vi "Register gRPC Methods.vi"(8 "error in (no error)":errorcluster, 11 "gRPC service in":refnum<class "Manager.lvclass">) -> (0 "error out":errorcluster, 3 "gRPC service out":refnum<class "Manager.lvclass">)   [LabVIEW 2021, in "CIF_Manager_server.lvlib" / "Manager.lvclass"]
uses:
  Manager.lvclass
  typeDefs/Server Internal UEs.ctl
  typeDefs/Server Internal Message.ctl
  typeDefs/Server gRPC UEs.ctl
  <vilib>/gRPC/LabVIEW gRPC Library/Server API/typeDefs/gRPCId Cluster.ctl
  <vilib>/gRPC/LabVIEW gRPC Library/Shared/grpcId.ctl
  Manager.lvclass/Manager.ctl
  <vilib>/gRPC/LabVIEW gRPC Library/grpc-lvsupport-release.lvlib
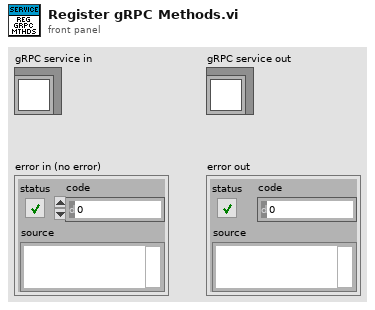
[diagram p1: front panel]
types:
  T1 = typedef "CIF_Manager_server.lvlib/Manager.lvclass/Server gRPC UEs.ctl" = cluster{"Manager LoadPlugin gRPC UE":refnum<user-event>, "Manager RegisterPlugin gRPC UE":refnum<user-event>, "Manager UnregisterPlugin gRPC UE":refnum<user-event>, "Manager QueryPluginTypes gRPC UE":refnum<user-event>, "Manager AbortPlugin gRPC UE":refnum<user-event>, "Manager UnloadAllPlugins gRPC UE":refnum<user-event>, "Manager Destroy gRPC UE":refnum<user-event>, "Manager Ping gRPC UE":refnum<user-event>, "Manager QueryErrors gRPC UE":refnum<user-event>, "Manager QueryConfig gRPC UE":refnum<user-event>, "Manager QueryInfo gRPC UE":refnum<user-event>, "Manager ResetErrorIndex gRPC UE":refnum<user-event>, "Manager ResetConfigIndex gRPC UE":refnum<user-event>, "Manager ResetInfoIndex gRPC UE":refnum<user-event>, "Manager QueryPluginInfo gRPC UE":refnum<user-event>, "Manager QueryPlugin gRPC UE":refnum<user-event>, "Manager QuerySystemStatus gRPC UE":refnum<user-event>, "Manager UpdateClock gRPC UE":refnum<user-event>, "Manager CreateOrch gRPC UE":refnum<user-event>, "Manager QueryClockStatus gRPC UE":refnum<user-event>, "Manager QueryAllChannels gRPC UE":refnum<user-event>, "Manager RegisterPluginLoader gRPC UE":refnum<user-event>, "Manager UnregisterPluginLoader gRPC UE":refnum<user-event>, "Manager CreatePluginLoader gRPC UE":refnum<user-event>, "Manager DestroyPluginLoader gRPC UE":refnum<user-event>, "Manager QueryPluginLoaders gRPC UE":refnum<user-event>}
  T2 = typedef "CIF_Manager_server.lvlib/Manager.lvclass/Server Internal UEs.ctl" = cluster{"Manager LoadPlugin Internal UE":refnum<user-event>, "Manager RegisterPlugin Internal UE":refnum<user-event>, "Manager UnregisterPlugin Internal UE":refnum<user-event>, "Manager QueryPluginTypes Internal UE":refnum<user-event>, "Manager AbortPlugin Internal UE":refnum<user-event>, "Manager UnloadAllPlugins Internal UE":refnum<user-event>, "Manager Destroy Internal UE":refnum<user-event>, "Manager Ping Internal UE":refnum<user-event>, "Manager QueryErrors Internal UE":refnum<user-event>, "Manager QueryConfig Internal UE":refnum<user-event>, "Manager QueryInfo Internal UE":refnum<user-event>, "Manager ResetErrorIndex Internal UE":refnum<user-event>, "Manager ResetConfigIndex Internal UE":refnum<user-event>, "Manager ResetInfoIndex Internal UE":refnum<user-event>, "Manager QueryPluginInfo Internal UE":refnum<user-event>, "Manager QueryPlugin Internal UE":refnum<user-event>, "Manager QuerySystemStatus Internal UE":refnum<user-event>, "Manager UpdateClock Internal UE":refnum<user-event>, "Manager CreateOrch Internal UE":refnum<user-event>, "Manager QueryClockStatus Internal UE":refnum<user-event>, "Manager QueryAllChannels Internal UE":refnum<user-event>, "Manager RegisterPluginLoader Internal UE":refnum<user-event>, "Manager UnregisterPluginLoader Internal UE":refnum<user-event>, "Manager CreatePluginLoader Internal UE":refnum<user-event>, "Manager DestroyPluginLoader Internal UE":refnum<user-event>, "Manager QueryPluginLoaders Internal UE":refnum<user-event>}
  T3 = typedef "grpc-lvsupport-release.lvlib/grpcId.ctl" = u64
  T4 = typedef "CIF_Manager_server.lvlib/Manager.lvclass/Server Internal Message UE.ctl" = refnum<user-event>
  T5 = typedef "grpc-lvsupport-release.lvlib/gRPCId Cluster UE.ctl" = refnum<user-event>
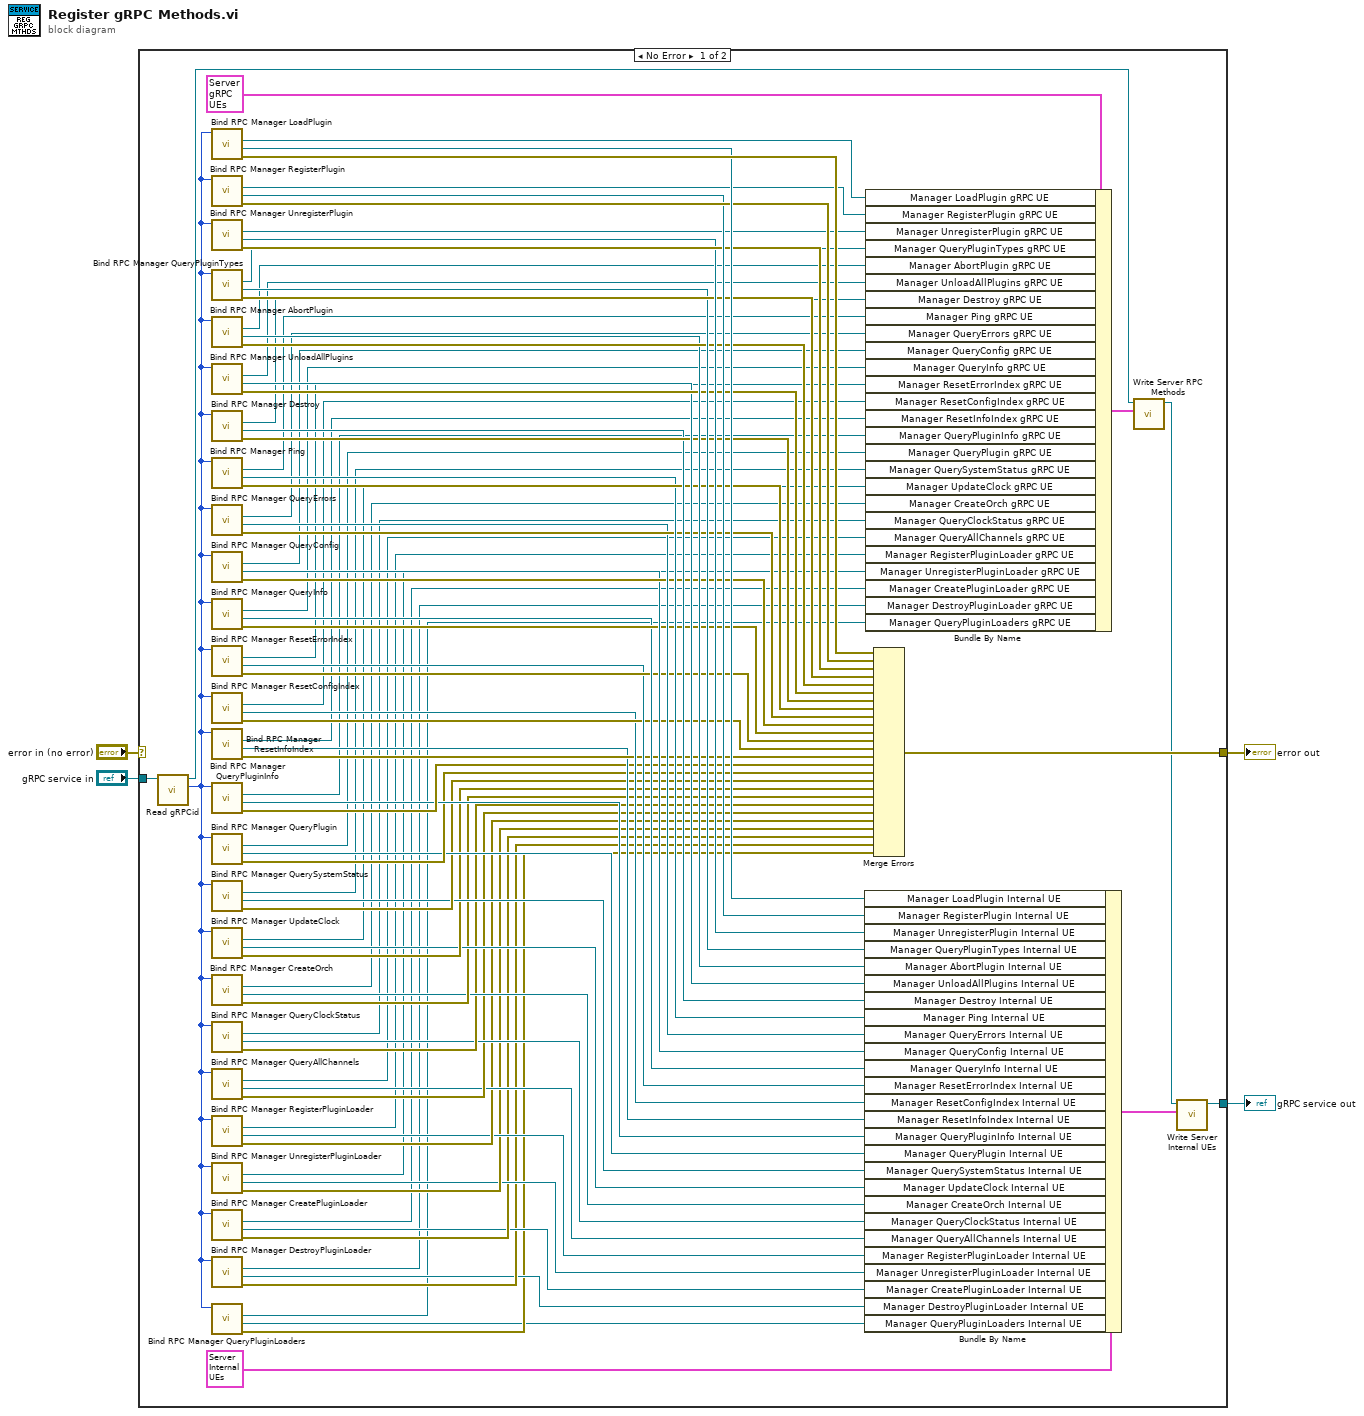
[diagram p0: block diagram]
diagram:
  n1 = case shown="No Error" "error in (no error)" {
    selector: "error in (no error)" -> [_ w93]
    tunnel: "gRPC service in" -> [w84 w94]
    tunnel: [w92 w93] -> w3
    tunnel: [w91 w94] -> w2
    frame No Error {
      n2 = call-dynamic "Read gRPCid.vi"("gRPC service in"=w84) -> ("gRPCid"=w83:T3, "gRPC service out"=w85:refnum<class "Manager.lvclass">)  [unwired: 8 in, 1 out]
      n3 = call "Bind RPC Manager LoadPlugin.vi"("gRPCid server in"=w83) -> ("error out"=w82:errorcluster, "Manager LoadPlugin Internal UE"=w81:T4, "Manager LoadPlugin gRPC UE"=w80:T5)  [unwired: 7 in, 1 out]
      n4 = call "Bind RPC Manager RegisterPlugin.vi"("gRPCid server in"=w83) -> ("error out"=w79:errorcluster, "Manager RegisterPlugin Internal UE"=w77:T4, "Manager RegisterPlugin gRPC UE"=w78:T5)  [unwired: 7 in, 1 out]
      n5 = call "Bind RPC Manager UnregisterPlugin.vi"("gRPCid server in"=w83) -> ("error out"=w76:errorcluster, "Manager UnregisterPlugin Internal UE"=w75:T4, "Manager UnregisterPlugin gRPC UE"=w74:T5)  [unwired: 7 in, 1 out]
      n6 = call "Bind RPC Manager QueryPluginTypes.vi"("gRPCid server in"=w83) -> ("error out"=w73:errorcluster, "Manager QueryPluginTypes Internal UE"=w71:T4, "Manager QueryPluginTypes gRPC UE"=w72:T5)  [unwired: 7 in, 1 out]
      n7 = call "Bind RPC Manager AbortPlugin.vi"("gRPCid server in"=w83) -> ("error out"=w70:errorcluster, "Manager AbortPlugin Internal UE"=w69:T4, "Manager AbortPlugin gRPC UE"=w68:T5)  [unwired: 7 in, 1 out]
      n8 = call "Bind RPC Manager UnloadAllPlugins.vi"("gRPCid server in"=w83) -> ("error out"=w67:errorcluster, "Manager UnloadAllPlugins Internal UE"=w65:T4, "Manager UnloadAllPlugins gRPC UE"=w66:T5)  [unwired: 7 in, 1 out]
      n9 = call "Bind RPC Manager Destroy.vi"("gRPCid server in"=w83) -> ("error out"=w64:errorcluster, "Manager Destroy Internal UE"=w63:T4, "Manager Destroy gRPC UE"=w62:T5)  [unwired: 7 in, 1 out]
      n10 = call "Bind RPC Manager Ping.vi"("gRPCid server in"=w83) -> ("error out"=w61:errorcluster, "Manager Ping Internal UE"=w59:T4, "Manager Ping gRPC UE"=w60:T5)  [unwired: 7 in, 1 out]
      n11 = call "Bind RPC Manager QueryErrors.vi"("gRPCid server in"=w83) -> ("error out"=w58:errorcluster, "Manager QueryErrors Internal UE"=w56:T4, "Manager QueryErrors gRPC UE"=w57:T5)  [unwired: 7 in, 1 out]
      n12 = call "Bind RPC Manager QueryConfig.vi"("gRPCid server in"=w83) -> ("error out"=w55:errorcluster, "Manager QueryConfig Internal UE"=w53:T4, "Manager QueryConfig gRPC UE"=w54:T5)  [unwired: 7 in, 1 out]
      n13 = call "Bind RPC Manager QueryInfo.vi"("gRPCid server in"=w83) -> ("error out"=w52:errorcluster, "Manager QueryInfo Internal UE"=w50:T4, "Manager QueryInfo gRPC UE"=w51:T5)  [unwired: 7 in, 1 out]
      n14 = call "Bind RPC Manager ResetErrorIndex.vi"("gRPCid server in"=w83) -> ("error out"=w49:errorcluster, "Manager ResetErrorIndex Internal UE"=w47:T4, "Manager ResetErrorIndex gRPC UE"=w48:T5)  [unwired: 7 in, 1 out]
      n15 = call "Bind RPC Manager ResetConfigIndex.vi"("gRPCid server in"=w83) -> ("error out"=w46:errorcluster, "Manager ResetConfigIndex Internal UE"=w44:T4, "Manager ResetConfigIndex gRPC UE"=w45:T5)  [unwired: 7 in, 1 out]
      n16 = call "Bind RPC Manager ResetInfoIndex.vi"("gRPCid server in"=w83) -> ("error out"=w43:errorcluster, "Manager ResetInfoIndex Internal UE"=w41:T4, "Manager ResetInfoIndex gRPC UE"=w42:T5)  [unwired: 7 in, 1 out]
      n17 = call "Bind RPC Manager QueryPluginInfo.vi"("gRPCid server in"=w83) -> ("error out"=w40:errorcluster, "Manager QueryPluginInfo Internal UE"=w39:T4, "Manager QueryPluginInfo gRPC UE"=w38:T5)  [unwired: 7 in, 1 out]
      n18 = call "Bind RPC Manager QueryPlugin.vi"("gRPCid server in"=w83) -> ("error out"=w37:errorcluster, "Manager QueryPlugin Internal UE"=w36:T4, "Manager QueryPlugin gRPC UE"=w35:T5)  [unwired: 7 in, 1 out]
      n19 = call "Bind RPC Manager QuerySystemStatus.vi"("gRPCid server in"=w83) -> ("error out"=w34:errorcluster, "Manager QuerySystemStatus Internal UE"=w32:T4, "Manager QuerySystemStatus gRPC UE"=w33:T5)  [unwired: 7 in, 1 out]
      n20 = call "Bind RPC Manager UpdateClock.vi"("gRPCid server in"=w83) -> ("error out"=w31:errorcluster, "Manager UpdateClock Internal UE"=w29:T4, "Manager UpdateClock gRPC UE"=w30:T5)  [unwired: 7 in, 1 out]
      n21 = call "Bind RPC Manager CreateOrch.vi"("gRPCid server in"=w83) -> ("error out"=w28:errorcluster, "Manager CreateOrch Internal UE"=w26:T4, "Manager CreateOrch gRPC UE"=w27:T5)  [unwired: 7 in, 1 out]
      n22 = call "Bind RPC Manager QueryClockStatus.vi"("gRPCid server in"=w83) -> ("error out"=w25:errorcluster, "Manager QueryClockStatus Internal UE"=w23:T4, "Manager QueryClockStatus gRPC UE"=w24:T5)  [unwired: 7 in, 1 out]
      n23 = call "Bind RPC Manager QueryAllChannels.vi"("gRPCid server in"=w83) -> ("error out"=w22:errorcluster, "Manager QueryAllChannels Internal UE"=w20:T4, "Manager QueryAllChannels gRPC UE"=w21:T5)  [unwired: 7 in, 1 out]
      n24 = call "Bind RPC Manager RegisterPluginLoader.vi"("gRPCid server in"=w83) -> ("error out"=w19:errorcluster, "Manager RegisterPluginLoader Internal UE"=w17:T4, "Manager RegisterPluginLoader gRPC UE"=w18:T5)  [unwired: 7 in, 1 out]
      n25 = call "Bind RPC Manager UnregisterPluginLoader.vi"("gRPCid server in"=w83) -> ("error out"=w16:errorcluster, "Manager UnregisterPluginLoader Internal UE"=w14:T4, "Manager UnregisterPluginLoader gRPC UE"=w15:T5)  [unwired: 7 in, 1 out]
      n26 = call "Bind RPC Manager CreatePluginLoader.vi"("gRPCid server in"=w83) -> ("error out"=w13:errorcluster, "Manager CreatePluginLoader Internal UE"=w11:T4, "Manager CreatePluginLoader gRPC UE"=w12:T5)  [unwired: 7 in, 1 out]
      n27 = call "Bind RPC Manager DestroyPluginLoader.vi"("gRPCid server in"=w83) -> ("error out"=w10:errorcluster, "Manager DestroyPluginLoader Internal UE"=w8:T4, "Manager DestroyPluginLoader gRPC UE"=w9:T5)  [unwired: 7 in, 1 out]
      n28 = call "Bind RPC Manager QueryPluginLoaders.vi"("gRPCid server in"=w83) -> ("error out"=w7:errorcluster, "Manager QueryPluginLoaders Internal UE"=w5:T4, "Manager QueryPluginLoaders gRPC UE"=w6:T5)  [unwired: 7 in, 1 out]
      n29 = Bundle By Name ("Bundle Internal UEs")(cluster=T2 {"Manager LoadPlugin Internal UE"=refnum, "Manager RegisterPlugin Internal UE"=refnum, "Manager UnregisterPlugin Internal UE"=refnum, "Manager QueryPluginTypes Internal UE"=refnum, "Manager AbortPlugin Internal UE"=refnum, "Manager UnloadAllPlugins Internal UE"=refnum, "Manager Destroy Internal UE"=refnum, "Manager Ping Internal UE"=refnum, "Manager QueryErrors Internal UE"=refnum, "Manager QueryConfig Internal UE"=refnum, "Manager QueryInfo Internal UE"=refnum, "Manager ResetErrorIndex Internal UE"=refnum, "Manager ResetConfigIndex Internal UE"=refnum, "Manager ResetInfoIndex Internal UE"=refnum, "Manager QueryPluginInfo Internal UE"=refnum, "Manager QueryPlugin Internal UE"=refnum, "Manager QuerySystemStatus Internal UE"=refnum, "Manager UpdateClock Internal UE"=refnum, "Manager CreateOrch Internal UE"=refnum, "Manager QueryClockStatus Internal UE"=refnum, "Manager QueryAllChannels Internal UE"=refnum, "Manager RegisterPluginLoader Internal UE"=refnum, "Manager UnregisterPluginLoader Internal UE"=refnum, "Manager CreatePluginLoader Internal UE"=refnum, "Manager DestroyPluginLoader Internal UE"=refnum, "Manager QueryPluginLoaders Internal UE"=refnum} ("Server Internal UEs"), "Manager LoadPlugin Internal UE"=w81, "Manager RegisterPlugin Internal UE"=w77, "Manager UnregisterPlugin Internal UE"=w75, "Manager QueryPluginTypes Internal UE"=w71, "Manager AbortPlugin Internal UE"=w69, "Manager UnloadAllPlugins Internal UE"=w65, "Manager Destroy Internal UE"=w63, "Manager Ping Internal UE"=w59, "Manager QueryErrors Internal UE"=w56, "Manager QueryConfig Internal UE"=w53, "Manager QueryInfo Internal UE"=w50, "Manager ResetErrorIndex Internal UE"=w47, "Manager ResetConfigIndex Internal UE"=w44, "Manager ResetInfoIndex Internal UE"=w41, "Manager QueryPluginInfo Internal UE"=w39, "Manager QueryPlugin Internal UE"=w36, "Manager QuerySystemStatus Internal UE"=w32, "Manager UpdateClock Internal UE"=w29, "Manager CreateOrch Internal UE"=w26, "Manager QueryClockStatus Internal UE"=w23, "Manager QueryAllChannels Internal UE"=w20, "Manager RegisterPluginLoader Internal UE"=w17, "Manager UnregisterPluginLoader Internal UE"=w14, "Manager CreatePluginLoader Internal UE"=w11, "Manager DestroyPluginLoader Internal UE"=w8, "Manager QueryPluginLoaders Internal UE"=w5) -> (w90:T2)
      n30 = Bundle By Name ("Bundle gRPC UEs")(cluster=T1 {"Manager LoadPlugin gRPC UE"=refnum, "Manager RegisterPlugin gRPC UE"=refnum, "Manager UnregisterPlugin gRPC UE"=refnum, "Manager QueryPluginTypes gRPC UE"=refnum, "Manager AbortPlugin gRPC UE"=refnum, "Manager UnloadAllPlugins gRPC UE"=refnum, "Manager Destroy gRPC UE"=refnum, "Manager Ping gRPC UE"=refnum, "Manager QueryErrors gRPC UE"=refnum, "Manager QueryConfig gRPC UE"=refnum, "Manager QueryInfo gRPC UE"=refnum, "Manager ResetErrorIndex gRPC UE"=refnum, "Manager ResetConfigIndex gRPC UE"=refnum, "Manager ResetInfoIndex gRPC UE"=refnum, "Manager QueryPluginInfo gRPC UE"=refnum, "Manager QueryPlugin gRPC UE"=refnum, "Manager QuerySystemStatus gRPC UE"=refnum, "Manager UpdateClock gRPC UE"=refnum, "Manager CreateOrch gRPC UE"=refnum, "Manager QueryClockStatus gRPC UE"=refnum, "Manager QueryAllChannels gRPC UE"=refnum, "Manager RegisterPluginLoader gRPC UE"=refnum, "Manager UnregisterPluginLoader gRPC UE"=refnum, "Manager CreatePluginLoader gRPC UE"=refnum, "Manager DestroyPluginLoader gRPC UE"=refnum, "Manager QueryPluginLoaders gRPC UE"=refnum} ("gRPC Server Method Events"), "Manager LoadPlugin gRPC UE"=w80, "Manager RegisterPlugin gRPC UE"=w78, "Manager UnregisterPlugin gRPC UE"=w74, "Manager QueryPluginTypes gRPC UE"=w72, "Manager AbortPlugin gRPC UE"=w68, "Manager UnloadAllPlugins gRPC UE"=w66, "Manager Destroy gRPC UE"=w62, "Manager Ping gRPC UE"=w60, "Manager QueryErrors gRPC UE"=w57, "Manager QueryConfig gRPC UE"=w54, "Manager QueryInfo gRPC UE"=w51, "Manager ResetErrorIndex gRPC UE"=w48, "Manager ResetConfigIndex gRPC UE"=w45, "Manager ResetInfoIndex gRPC UE"=w42, "Manager QueryPluginInfo gRPC UE"=w38, "Manager QueryPlugin gRPC UE"=w35, "Manager QuerySystemStatus gRPC UE"=w33, "Manager UpdateClock gRPC UE"=w30, "Manager CreateOrch gRPC UE"=w27, "Manager QueryClockStatus gRPC UE"=w24, "Manager QueryAllChannels gRPC UE"=w21, "Manager RegisterPluginLoader gRPC UE"=w18, "Manager UnregisterPluginLoader gRPC UE"=w15, "Manager CreatePluginLoader gRPC UE"=w12, "Manager DestroyPluginLoader gRPC UE"=w9, "Manager QueryPluginLoaders gRPC UE"=w6) -> (w87:T1)
      n31 = Merge Errors(w82, w79, w76, w73, w70, w67, w64, w61, w58, w55, w52, w49, w46, w43, w40, w37, w34, w31, w28, w25, w22, w19, w16, w13, w10, w7) -> (w92:errorcluster)
      n32 = call "Write Server RPC Methods.vi"("Server RPC Methods"=w87, "gRPC service in"=w85) -> ("gRPC service out"=w88:refnum<class "Manager.lvclass">)  [unwired: 8 in, 1 out]
      n33 = call "Write Server Internal UEs.vi"("Server Internal UEs"=w90, "gRPC service in"=w88) -> ("gRPC service out"=w91:refnum<class "Manager.lvclass">)  [unwired: 8 in, 1 out]
    }
    frame Error {
    }
  }
  "error out" <- w3
  "gRPC service out" <- w2
